vi "Fdx Read Monitor Queue.vi"(6 "MaxReadBytes":u32=65536, 7 "ReadQualifier (0:full)":u32, 8 "error in (no error)":errorcluster, 9 "EntryCount (1)":u32=1, 10 "QueueId in":u32, 11 "InstrumentHandle_port in":u32) -> (0 "error out":errorcluster, 1 "QueueReadOut":T1, 2 "QueueId out":u32, 3 "InstrumentHandle_port out":u32)   [LabVIEW 2020, in "AIM664LV.lvlib"]
uses:
  AIM664LV.lvlib
panel:
  # "/* FdxCmdMonQueueRead*/\n#define FDX_MON_READ_FULL              0\n#define FDX_MON_READ_HEADER            1\n#define FDX_MON_READ_DATA              2"
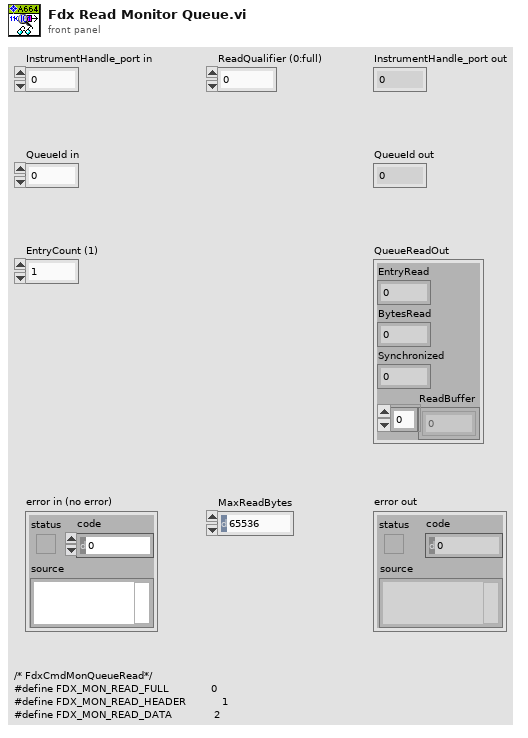
[diagram p1: front panel]
types:
  T1 = cluster{"EntryRead":u32, "BytesRead":u32, "Synchronized":u32, "ReadBuffer":u8[]}
  T2 = cluster{"QueueId":u32, "EntryCount":u32, "ReadQualifier":u32, "MaxReadBytes":u32}
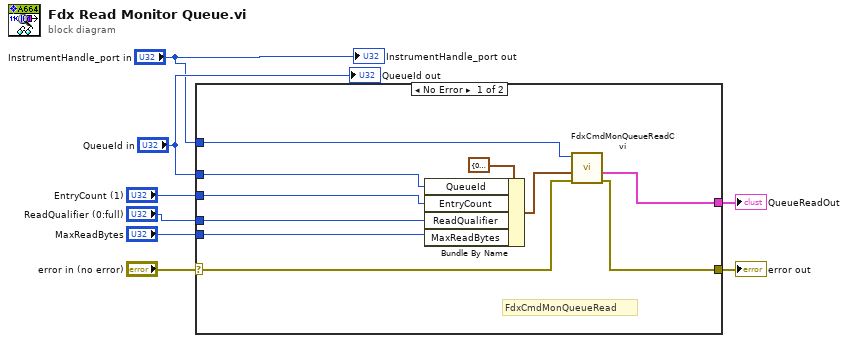
[diagram p0: block diagram]
diagram:
  n1 = case shown="No Error" "error in (no error)" {
    selector: "error in (no error)" -> [w18 w19]
    tunnel: [w15 w19] -> w7
    tunnel: "InstrumentHandle_port in" -> [w9 _]
    tunnel: [w14 _] -> w6
    tunnel: "EntryCount (1)" -> [w13 _]
    tunnel: "ReadQualifier (0:full)" -> [w12 _]
    tunnel: "MaxReadBytes" -> [w11 _]
    tunnel: "QueueId in" -> [w10 _]
    frame No Error {
      # "FdxCmdMonQueueRead"
      n2 = Bundle By Name(cluster=T2 {"QueueId"=0, "EntryCount"=0, "ReadQualifier"=0, "MaxReadBytes"=0} ("QueueReadIn"), "QueueId"=w10, "EntryCount"=w13, "ReadQualifier"=w12, "MaxReadBytes"=w11) -> (w16:T2)
      n3 = call "FdxCmdMonQueueReadCvi.vi"("error in"=w18, "QueueReadIn"=w16, "InstrumentHandle_port"=w9) -> ("error out"=w15:errorcluster, "QueueReadOut"=w14:T1)  [unwired: 6 in, 1 out]
    }
    frame Error {
    }
  }
  "error out" <- w7
  "QueueReadOut" <- w6
  "InstrumentHandle_port out" <- "InstrumentHandle_port in"
  "QueueId out" <- "QueueId in"
